vi "9401_Initialize.vi"(8 "error in (no error)":errorcluster, 9 "Slot Settings":T1, 11 "9401 in":refnum<class "9401.lvclass">) -> (0 "error out":errorcluster, 3 "9401 out":refnum<class "9401.lvclass">)   [LabVIEW 2019, in "Modules.lvlib" / "9401.lvclass"]
uses:
  9401.lvclass
  RSI Module/Slot Settings.ctl
  C:/Users/nitest/Desktop/Git 2019/niveristand-scan-engine-module-libraries/Source/SD Module/SD Module.lvclass
  C:/Users/nitest/Desktop/Git 2019/niveristand-scan-engine-module-libraries/Source/RSI Module/RSI Module.lvclass
  RSI Module/Channels.ctl
  RSI Module/Channel Type.ctl
  RSI Module/Module Models.ctl
  9401.lvclass/9401.ctl
  RSI Module/RSI Module.lvclass
  SD Module/SD Module.lvclass
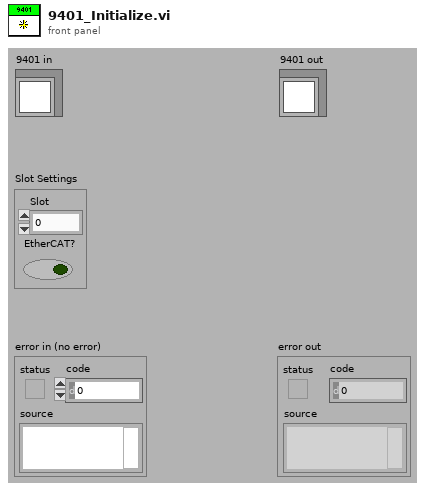
[diagram p1: front panel]
types:
  T1 = typedef "Modules.lvlib/RSI Module.lvclass/Slot Settings.ctl" = cluster{"Slot":u32, "EtherCAT?":bool}
  T2 = typedef "Modules.lvlib/RSI Module.lvclass/Module Models.ctl" = enum16{"Empty", "NI 9201", "NI 9203", "NI 9205", "NI 9206", "NI 9207", "NI 9208", "NI 9209", "NI 9210", "NI 9211", "NI 9212", "NI 9213", "NI 9214", "NI 9215", "NI 9216", "NI 9217", "NI 9219", "NI 9220", "NI 9221", "NI 9222", "NI 9223", "NI 9224", "NI 9225", "NI 9226", "NI 9227", "NI 9228", "NI 9229", "NI 9233", "NI 9234", "NI 9235", "NI 9236", "NI 9237", "NI 9239", "NI 9242", "NI 9244", "NI 9253", "NI 9263", "NI 9264", "NI 9265", "NI 9266", "NI 9269", "NI 9344", "NI 9350", "NI 9375", "NI 9401", "NI 9402", "NI 9403", "NI 9411", "NI 9421", "NI 9422", "NI 9423", "NI 9425", "NI 9426", "NI 9435", "NI 9436", "NI 9437", "NI 9472", "NI 9474", "NI 9475", "NI 9476", "NI 9477", "NI 9478", "NI 9481", "NI 9482", "NI 9485"}
  T3 = typedef "Modules.lvlib/RSI Module.lvclass/Channels.ctl" = cluster{"# Input Channels":i32, "# Output Channels":i32, "Channel Type":T4, "Units":string}
  T4 = typedef "Modules.lvlib/RSI Module.lvclass/Channel Type.ctl" = enum16{"Analog", "Digital"}
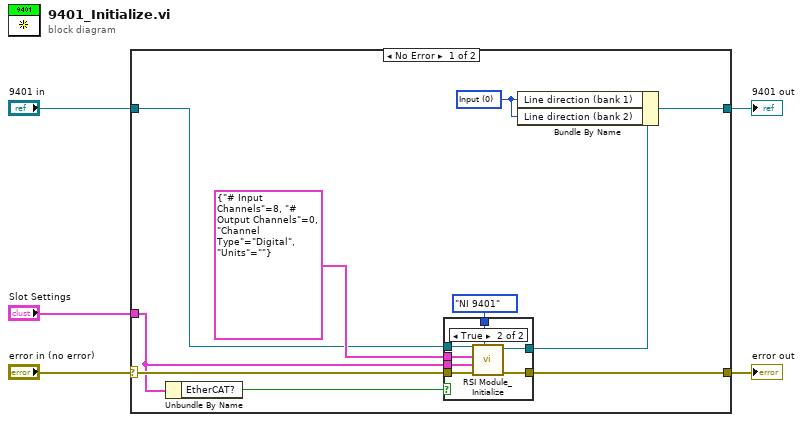
[diagram p0: block diagram]
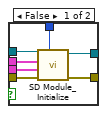
[diagram p2: hidden frame]
diagram:
  n1 = case shown="No Error" "error in (no error)" {
    selector: "error in (no error)" -> [w13 w31]
    tunnel: [w12 w31] -> w4
    tunnel: [w10 w30] -> w2
    tunnel: "9401 in" -> [w14 w30]
    tunnel: "Slot Settings" -> [w8 _]
    frame No Error {
      w9 = u32 0 items=["Input", "Output"] ("Line direction (bank 1)")
      n2 = Unbundle By Name(w8) -> ("EtherCAT?"=w7:bool)
      n3 = case shown="True" w7 {
        tunnel: T3 {"# Input Channels"=8, "# Output Channels"=0, "Channel Type"=enum."Digital", "Units"=""} ("Channels") -> [w22 w23]
        tunnel: w14 -> [w21 w26]
        tunnel: w8 -> [w20 w24]
        tunnel: w13 -> [w19 w25]
        tunnel: [w18 w27] -> w12
        tunnel: [w17 w28] -> w11
        tunnel: Module_Models."NI 9401" ("Module Model") -> [w16 w29]
        frame False {
          n4 = call "SD Module_Initialize.vi"("Module Model"=w16, "error in (no error)"=w19, "Slot Settings"=w20, "Channels"=w22, "SD Module in"=w21) -> ("error out"=w18:errorcluster, "SD Module out"=w17:refnum<class "9401.lvclass">)  [unwired: 5 in]
        }
        frame True {
          n5 = call "RSI Module_Initialize.vi"("Module Model"=w29, "error in (no error)"=w25, "Slot Settings"=w24, "Channels"=w23, "RSI Module in"=w26) -> ("error out"=w27:errorcluster, "RSI Module out"=w28:refnum<class "9401.lvclass">)  [unwired: 5 in]
        }
      }
      n6 = Bundle By Name(cluster=w11, "Line direction (bank 1)"=w9, "Line direction (bank 2)"=w9) -> (w10:refnum<class "9401.lvclass">)
    }
    frame Error {
    }
  }
  "error out" <- w4
  "9401 out" <- w2
